vi "Process New Connection.vi"(8 "error in (no error)":errorcluster, 10 "Connection Reference":refnum<data-value>, 11 "New Connection Policy in":refnum<class "New Connection Policy.lvclass">) -> (0 "error out":errorcluster)   [LabVIEW 2019, in "PersitantConnectionHandler.lvlib" / "New Connection Policy.lvclass"]
uses:
  <vilib>/gpm_packages/@cs/Network-interface/Source/PersistantConnectionHandler/New Connection Policy/New Connection Policy.lvclass
  <vilib>/gpm_packages/@cs/Network-interface/Source/Connection Reference/Connection Reference/Connection Reference.lvclass
  <vilib>/gpm_packages/@cs/Network-interface/Source/PersistantConnectionHandler/New Connection Policy/New Connection Policy.lvclass/New Connection Policy.ctl
  <vilib>/gpm_packages/@cs/Network-interface/Source/PersistantConnectionHandler/PersistantConnectionHandler Messages/Process New Connection Msg/Process New Connection Msg.lvclass/Process New Connection Msg.ctl
  <vilib>/ActorFramework/Message Enqueuer/Message Enqueuer.lvclass/Message Enqueuer.ctl
  <vilib>/ActorFramework/Message Enqueuer/Enqueue.vi
  <vilib>/gpm_packages/@cs/Network-interface/Source/PersistantConnectionHandler/PersistantConnectionHandler Messages/Process New Connection Msg/Process New Connection Msg.lvclass
  C:/Program Files/National Instruments/LabVIEW 2019/vi.lib/ActorFramework/Message/Message.lvclass
  <vilib>/ActorFramework/Message Priority Queue/Priority Enqueue.vi
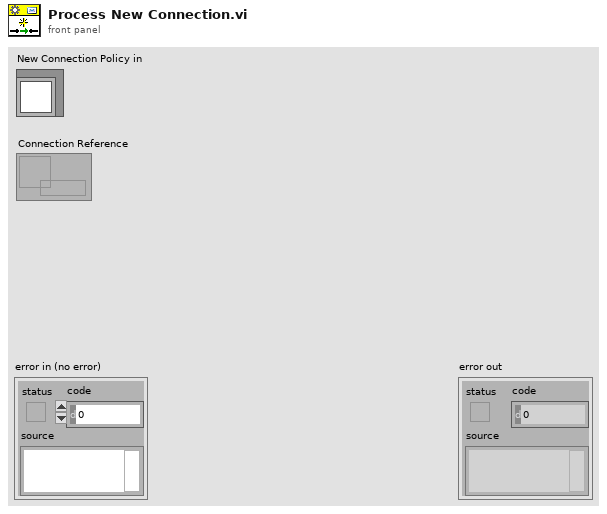
[diagram p1: front panel]
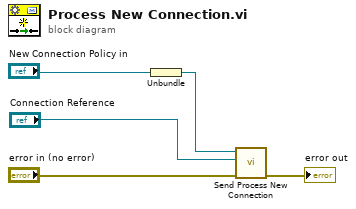
[diagram p0: block diagram]
diagram:
  n1 = Unbundle("New Connection Policy in") -> (w2:refnum<class "Message Enqueuer.lvclass">)
  n2 = call <vilib>:"Send Process New Connection.vi"("error in (no error)"="error in (no error)", "Connection Reference"="Connection Reference", "Message Enqueuer"=w2) -> ("error out"=→"error out":errorcluster)  [unwired: 7 in, 1 out]
